vi "Event Handler.vi"(8 "error in":errorcluster, 10 "Stop Event Handler":refnum<user-event>, 11 "EmailField in":refnum<class "EmailField.lvclass">) -> (0 "error out":errorcluster)   [LabVIEW 2020, in "EmailField.lvclass"]
doc: "The <b>Event Handler VI</b> is a dynamic dispatch VI that should be overwritten if events are needed to create the enhanced QControl. \n\nBy inheriting from the main Control.lvclass the overwritten <b>Event Handler VI</b> will be launched asynchronously in the initialization of the QControl.\n<b> </b> <b> </b>\n©2016 Q Software Innovations, LLC (QSI)\nwritten by Quentin Alldredge\nproduced in LabVIEW 2015\n\nsupport@qsoftwareinnovations.com\nwww.qsoftwareinnovations.com\n\nAll rights reserved.\n\nRedistribution and use in source and binary forms, with or without modification, are permitted provided that the following conditions are met:\n\n * Redistributions of source code must retain the above copyright notice, this list of conditions and the following disclaimer.\n * Redistributions in binary form must reproduce the above copyright notice, this list of conditions and the following disclaimer in the documentation and/or other materials provided with the distribution.\n * Neither the name of Q Software Innovations, LLC. nor the names of its contributors may be used to endorse or promote products derived from this software without specific prior written permission.\n\nTHIS SOFTWARE IS PROVIDED BY THE COPYRIGHT HOLDERS AND CONTRIBUTORS \"AS IS\" AND ANY EXPRESS OR IMPLIED WARRANTIES, INCLUDING, BUT NOT LIMITED TO, THE IMPLIED WARRANTIES OF MERCHANTABILITY AND FITNESS FOR A PARTICULAR PURPOSE ARE DISCLAIMED. IN NO EVENT SHALL THE COPYRIGHT OWNER OR CONTRIBUTORS BE LIABLE FOR ANY DIRECT, INDIRECT, INCIDENTAL, SPECIAL, EXEMPLARY, OR CONSEQUENTIAL DAMAGES (INCLUDING, BUT NOT LIMITED TO, PROCUREMENT OF SUBSTITUTE GOODS OR SERVICES; LOSS OF USE, DATA, OR PROFITS; OR BUSINESS INTERRUPTION) HOWEVER CAUSED AND ON ANY THEORY OF LIABILITY, WHETHER IN CONTRACT, STRICT LIABILITY, OR TORT (INCLUDING NEGLIGENCE OR OTHERWISE) ARISING IN ANY WAY OUT OF THE USE OF THIS SOFTWARE, EVEN IF ADVISED OF THE POSSIBILITY OF SUCH DAMAGE."
uses:
  EmailField.lvclass
  C:/Program Files (x86)/National Instruments/LabVIEW 2020/vi.lib/QSI/QControls/QControl Classes/String/String.lvclass
  EmailField.lvclass/EmailField.ctl
  Read ErrorColorBG.vi
  Read CorrectColorBG.vi
  Read ErrorColorText.vi
  Read CorrectColorText.vi
  <vilib>/regexp/Match Regular Expression.xnode
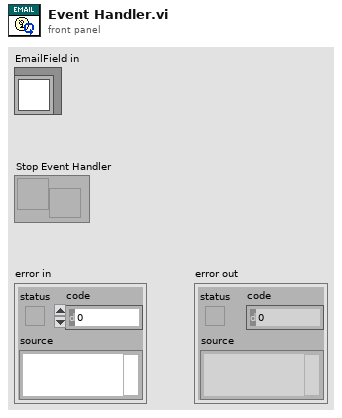
[diagram p1: front panel]
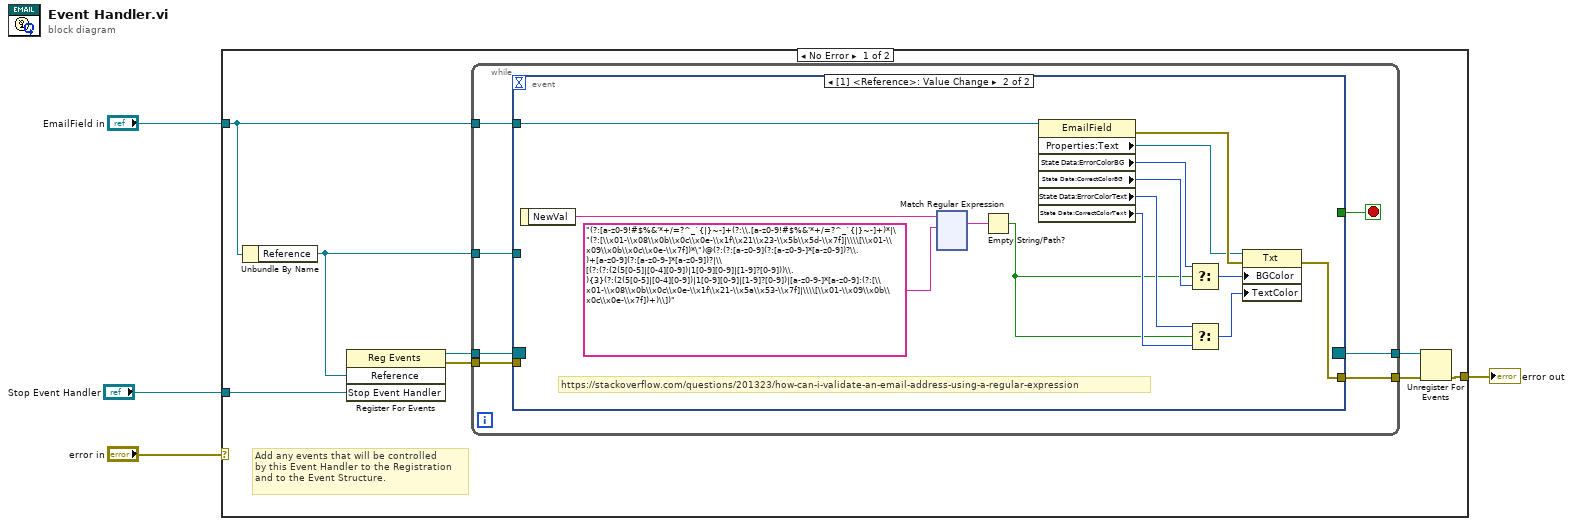
[diagram p0: block diagram]
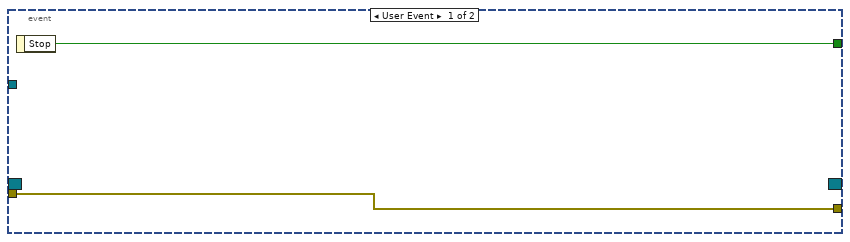
[diagram p2: hidden frame]
diagram:
  n1 = case shown="No Error" "error in" {
    selector: "error in" -> [_ w150]
    tunnel: [w10 w150] -> w3
    tunnel: "EmailField in" -> [w7 _]
    tunnel: "Stop Event Handler" -> [w5 _]
    frame No Error {
      # "Add any events that will be controlled\nby this Event Handler to the Registration\nand to the Event Structure."
      n2 = Unbundle By Name(w7) -> ("Reference"=w6:refnum<vi>)
      n3 = register-events(w6, w5) -> (reference out=w9:refnum<event-registration>, error out=w12:errorcluster)  [unwired: 2 in]
      n4 = while {
        tunnel: w9 -> [w17]
        tunnel: w12 -> [w19]
        tunnel: [w18] -> w11
        tunnel: [w14] -> w8
        tunnel: w6 -> [w13]
        tunnel: w7 -> [w16]
        stop <- w15 stop-if-true
        n5 = event shown="[1] <Reference>: Value Change" {
          selector: w17 -> [_ _]
          dyn-events: [_ _] -> w14
          timeout: _ -> [_ _]
          tunnel: w16 -> [_ w33]
          tunnel: w19 -> [w21 _]
          tunnel: [w21 w34] -> w18
          tunnel: [w20 _] -> w15
          tunnel: w13 -> [_ _]
          event User Event {
            n6 = event-data() -> ("Stop"=w20:bool)  [unwired: 1 in]
          }
          event Value Change {
            # "https://stackoverflow.com/questions/201323/how-can-i-validate-an-email-address-using-a-regular-expression"
            n7 = event-data() -> ("NewVal"=w32:string)  [unwired: 1 in]
            n8 = xnode "Match Regular Expression"("input string"=w32, "regular expression"="(?:[a-z0-9!#$%&'*+/=?^_`{|}~-]+(?:\\.[a-z0-9!#$%&'*+/=?^_`{|}~-]+)*|\"(?:[\\x01-\\x08\\x0b\\x0c\\x0e-\\x1f\\x21\\x23-\\x5b\\x5d-\\x7f]|\\\\[\\x01-\\x09\\x0b\\x0c\\x0e-\\x7f])*\")@(?:(?:[a-z0-9](?:[a-z0-9-]*[a-z0-9])?\\.)+[a-z0-9](?:[a-z0-9-]*[a-z0-9])?|\\[(?:(?:(2(5[0-5]|[0-4][0-9])|1[0-9][0-9]|[1-9]?[0-9]))\\.){3}(?:(2(5[0-5]|[0-4][0-9])|1[0-9][0-9]|[1-9]?[0-9])|[a-z0-9-]*[a-z0-9]:(?:[\\x01-\\x08\\x0b\\x0c\\x0e-\\x1f\\x21-\\x5a\\x53-\\x7f]|\\\\[\\x01-\\x09\\x0b\\x0c\\x0e-\\x7f])+)\\])") -> ("whole match"=w30:string)  [unwired: 4 in, 4 out]
            n9 = Empty String/Path?(string/path=w30) -> (empty?=w22:bool)
            n10 = property class="EmailField"(reference=w33) -> (error out=w35:errorcluster, "Properties:Text"=w31:refnum<vi>, "State Data:ErrorColorBG"=w24:u32, "State Data:CorrectColorBG"=w25:u32, "State Data:ErrorColorText"=w26:u32, "State Data:CorrectColorText"=w27:u32)  [unwired: 1 in, 1 out]
            n11 = Select(t=w24, s=w22, f=w25) -> (s? t:f=w29:u32)
            n12 = Select(t=w26, s=w22, f=w27) -> (s? t:f=w28:u32)
            n13 = property class="Txt"(reference=w31, error in=w35, "BGColor"=w29, "TextColor"=w28) -> (error out=w34:errorcluster)  [unwired: 1 out]
          }
        }
      }
      n14 = Unregister For Events(event registration refnum=w8, error in=w11) -> (error out=w10:errorcluster)
    }
    frame Error {
    }
  }
  "error out" <- w3
